vi "testDerivedKeyUniqueness.vi"(8 "error in (no error)":errorcluster, 11 "TestCase in":refnum<class "TestPBKDF2.lvclass">) -> (0 "error out":errorcluster, 3 "TestCase out":refnum<class "TestPBKDF2.lvclass">)   [LabVIEW 2021, in "TestPBKDF2.lvclass"]
uses:
  TestPBKDF2.lvclass
  Source Code/Asymmetric Encryption/RSA/HashingAlgorithm.ctl
  <vilib>/addons/_JKI Toolkits/VI Tester/TestCase.llb/TestCase.lvclass
  Source Code/Key Derivation/dotNET Crypto Key Derivation.lvlib
  Source Code/Utility/dotNET Crypto Utility.lvlib
  C:/Program Files (x86)/National Instruments/LabVIEW 2021/vi.lib/addons/_JKI Toolkits/VI Tester/TestCase.llb/TestCase.lvclass
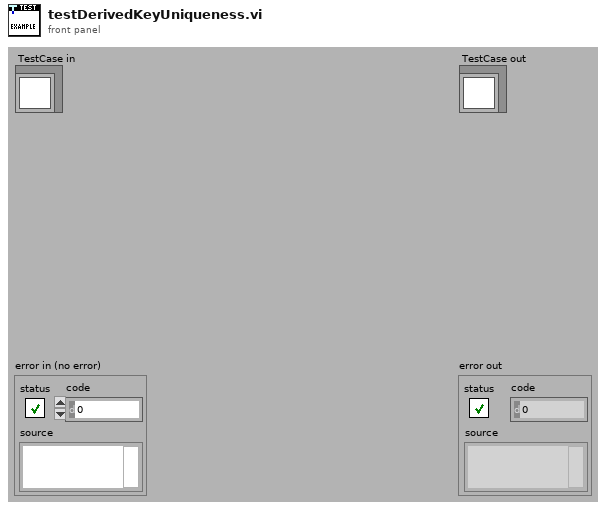
[diagram p1: front panel]
types:
  T1 = typedef "dotNET Crypto Utility.lvlib/HashingAlgorithm.ctl" = enum16{"MD5", "SHA1", "SHA256", "SHA384", "SHA512"}
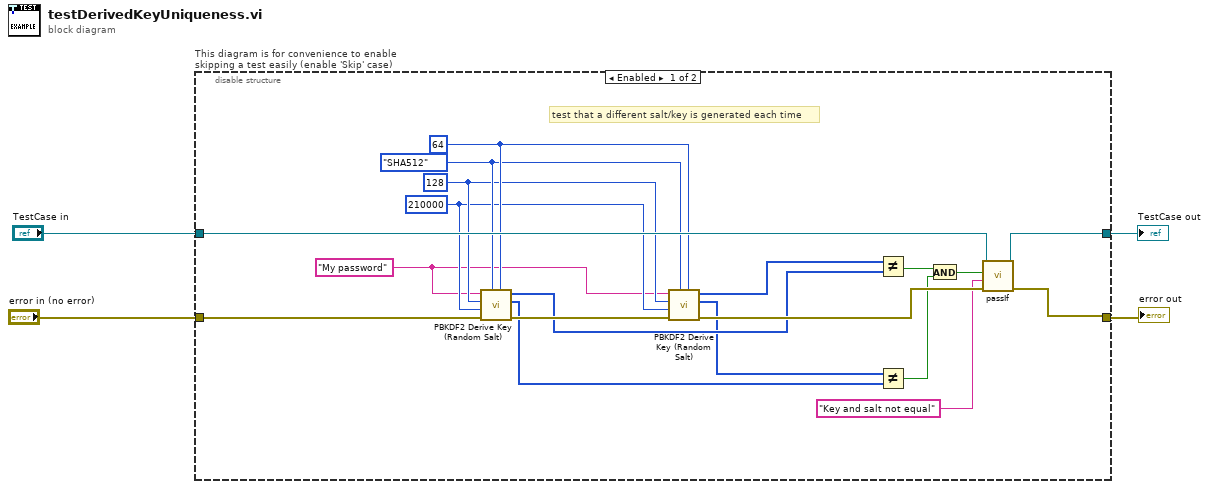
[diagram p0: block diagram]
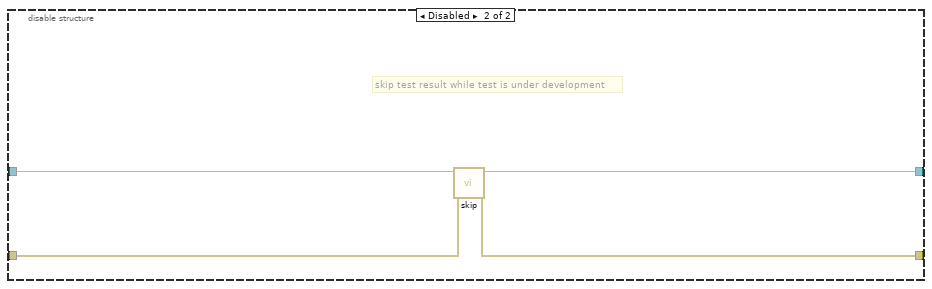
[diagram p2: hidden frame]
diagram:
  n1 = disable-structure "This diagram is for convenience to enable skipping a test easily (enable 'Skip' case)" shown="Enabled" {
    disable-tunnel: "TestCase in" -> [w23 w27]
    disable-tunnel: [w22 w25] -> w1
    disable-tunnel: [w21 w26] -> w3
    disable-tunnel: "error in (no error)" -> [w20 w24]
    frame Enabled {
      w13 = "My password" ("Password")
      w14 = 210000 ("iterations (210000)")
      w15 = 128 ("saltSize (128)")
      w16 = HashingAlgorithm."SHA512" ("HashingAlgorithm (SHA512)")
      w17 = 64 ("Key length (64 bytes)")
      # "test that a different salt/key is generated each time"
      n2 = call "PBKDF2 Derive Key (Random Salt).vi"("Key length (64 bytes)"=w17, "HashingAlgorithm (SHA512)"=w16, "error in (no error)"=w20, "iterations (210000)"=w14, "saltSize (16 bytes)"=w15, "Password"=w13) -> ("error out"=w19:errorcluster, "Salt"=w9:u8[], "Derived Key"=w11:u8[])  [unwired: 3 in]
      n3 = call "PBKDF2 Derive Key (Random Salt).vi"("Key length (64 bytes)"=w17, "HashingAlgorithm (SHA512)"=w16, "error in (no error)"=w19, "iterations (210000)"=w14, "saltSize (16 bytes)"=w15, "Password"=w13) -> ("error out"=w18:errorcluster, "Salt"=w10:u8[], "Derived Key"=w12:u8[])  [unwired: 3 in]
      n4 = Not Equal?(x=w12, y=w11) -> (x != y?=w8:bool)
      n5 = Not Equal?(x=w10, y=w9) -> (x != y?=w7:bool)
      n6 = And(x=w8, y=w7) -> (x .and. y?=w6:bool)
      n7 = call-dynamic "passIf.vi"("error in (no error)"=w18, "message (\"\")"="Key and salt not equal" ("message (\"\")"), "pass"=w6, "TestCase in"=w23) -> ("error out"=w21:errorcluster, "TestCase out"=w22:refnum<class "TestPBKDF2.lvclass">)  [unwired: 6 in]
    }
    frame Disabled {
      # "skip test result while test is under development"
      n8 = call <vilib>:"skip.vi"("error in (no error)"=w24, "TestCase in"=w27) -> ("error out"=w26:errorcluster, "TestCase out"=w25:refnum<class "TestPBKDF2.lvclass">)  [unwired: 8 in]
    }
  }
  "error out" <- w3
  "TestCase out" <- w1
